vi "RerangeCurrent.vi"(0 "XYGraph in":refnum<vi>, 3 "x":dbl, 5 "Cluster in":cluster{"Y":dbl[], "Current (A)":dbl[]}, 7 "SweepInfo":T1={"Current Range"=1e-10, "Source Measure Unit Channel (0: Channel A)"=0, "Waveform"={"t0"=timestamp(0 s since 1904-01-01), "dt"=1.0, "Y"=[]}, "VISA resource name"="", "CodeText"=""}, 9 "IVCurve in":dbl[][](array[numeric]), 12 "Fit 3":dbl[](array[numeric]), 14 "Rerange":bool) -> (4 "IVCurve":dbl[][](array[numeric]), 6 "Fit 2":dbl[](array[numeric]), 8 "Cluster out":cluster{"Y":dbl[], "Current (A)":dbl[]})   [LabVIEW 2020]
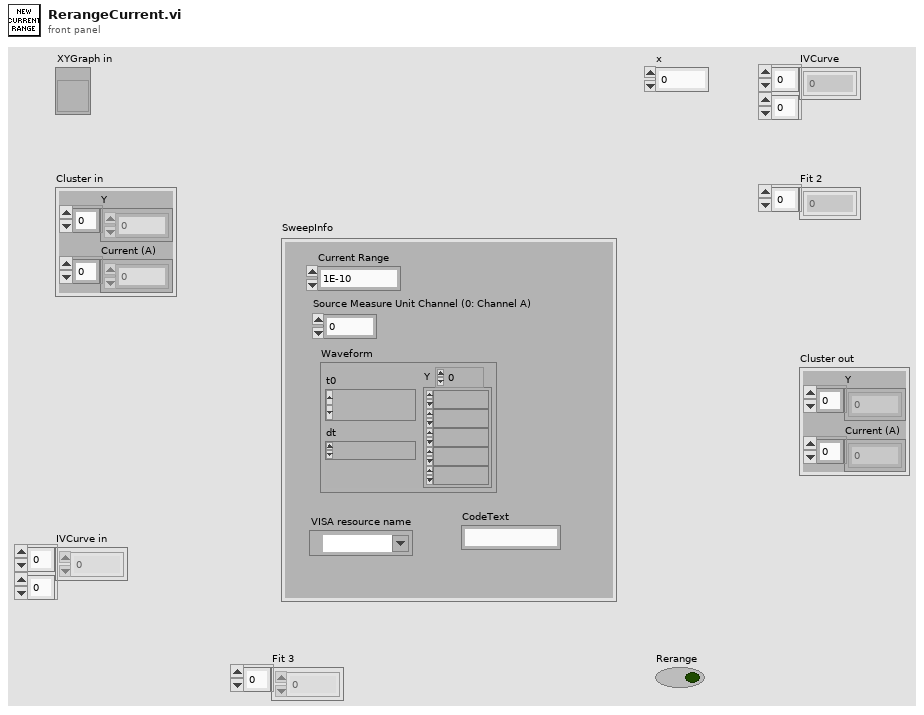
[diagram p1: front panel]
types:
  T1 = cluster{"Current Range":dbl, "Source Measure Unit Channel (0: Channel A)":i32, "Waveform":waveform(dbl), "VISA resource name":refnum<visa-resource-name>, "CodeText":string}
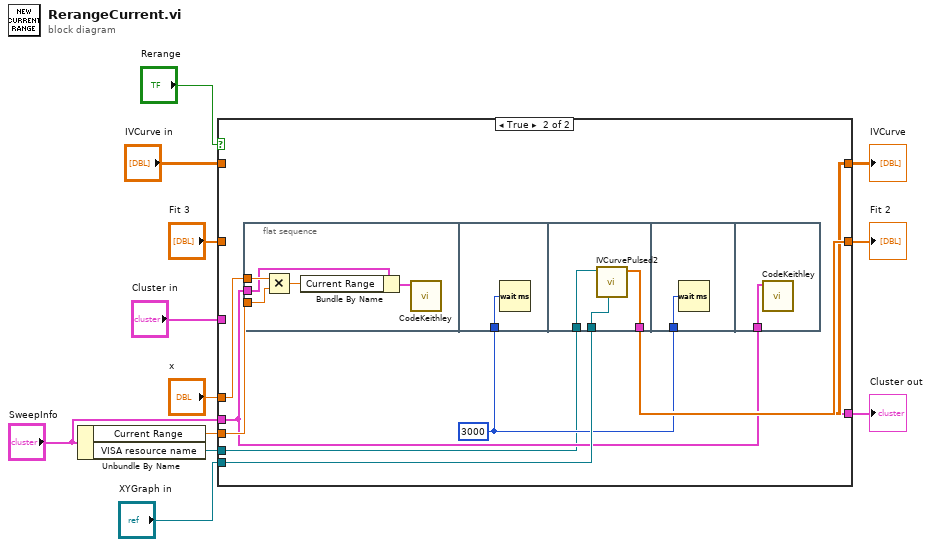
[diagram p0: block diagram]
diagram:
  n1 = Unbundle By Name("SweepInfo") -> ("Current Range"=w3:dbl, "VISA resource name"=w1:refnum<visa-resource-name>)
  n2 = case shown="True" "Rerange" {
    tunnel: [w15 w21] -> w6
    tunnel: "IVCurve in" -> [w15 _]
    tunnel: [w14 w22] -> w8
    tunnel: "Fit 3" -> [w14 _]
    tunnel: "XYGraph in" -> [_ w23]
    tunnel: [w13 w20] -> w11
    tunnel: "Cluster in" -> [w13 _]
    tunnel: w3 -> [_ w24]
    tunnel: "x" -> [_ w19]
    tunnel: "SweepInfo" -> [_ w17]
    tunnel: w1 -> [_ w16]
    frame False {
    }
    frame True {
      w18 = u32 3000 ("milliseconds to wait")
      n3 = flat-sequence {
        tunnel: w24 -> [w29]
        tunnel: w19 -> [w28]
        tunnel: w17 -> [w26]
        tunnel: w18 -> [w30]
        tunnel: w23 -> [w35]
        tunnel: [w34] -> w22
        tunnel: [w33] -> w21
        tunnel: [w32] -> w20
        tunnel: w16 -> [w31]
        tunnel: w18 -> [w36]
        tunnel: w17 -> [w37]
        frame #0 {
          n4 = Multiply(x=w28, y=w29) -> (x*y=w27:dbl)
          n5 = Bundle By Name(cluster=w26, "Current Range"=w27) -> (w25:T1)
          n6 = call "CodeKeithley.vi"("SweepInfo"=w25) -> ()  [unwired: 10 in, 1 out]
        }
        frame #1 {
          n7 = Wait (ms)(milliseconds to wait=w30) -> ()  [unwired: 1 out]
        }
        frame #2 {
          n8 = call "IVCurvePulsed2.vi"("XYGraph Refnum"=w35, "VISA Refnum in"=w31) -> ("Fit 2"=w34:dbl[], "appended array"=w33:dbl[][], "Cluster"=w32:cluster{"Y":dbl[], "Current (A)":dbl[]})  [unwired: 7 in]
        }
        frame #3 {
          n9 = Wait (ms)(milliseconds to wait=w36) -> ()  [unwired: 1 out]
        }
        frame #4 {
          n10 = call "CodeKeithley.vi"("SweepInfo"=w37) -> ()  [unwired: 10 in, 1 out]
        }
      }
    }
  }
  "Cluster out" <- w11
  "Fit 2" <- w8
  "IVCurve" <- w6
